vi "Launch CO2 Actor.vi"(4 "SHVs":cluster{"Halt":refnum<k21>}, 5 "DedicatedEnQrs":refnum<queue>, 6 "Open Actor Core front panel? (F)":bool, 7 "Name":string, 8 "error in (no error)":errorcluster, 9 "Interlock Chain":refnum<class "Interlock Chain.lvclass">, 10 "Caller Actor in":refnum<class "Actor.lvclass">, 11 "CO2 Actor in":refnum<class "CO2 Actor.lvclass">) -> (0 "error out":errorcluster, 3 "Caller-To-Actor Enqueuer":refnum<class "Message Enqueuer.lvclass">)   [LabVIEW 2015, in "cRIO-Carbondioxide.lvlib" / "CO2-Actor.lvlib" / "CO2 Actor.lvclass"]
uses:
  CO2 Actor.lvclass
  Interlocks/Interlock Chain/Interlock Chain.lvclass
  <vilib>/ActorFramework/Actor/Actor.lvclass
  <vilib>/ActorFramework/Message Enqueuer/Message Enqueuer.lvclass
  Controls/Dedicated Enqueuers.ctl
  CO2 Actor.lvclass/CO2 Actor.ctl
panel:
  out "CO2 Actor out":refnum<class "CO2 Actor.lvclass">
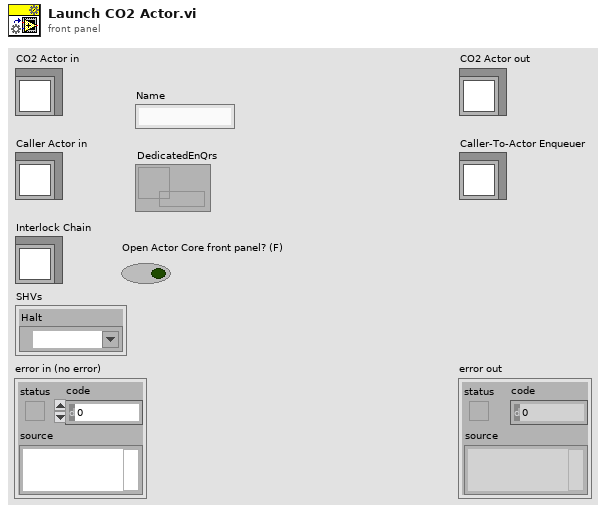
[diagram p1: front panel]
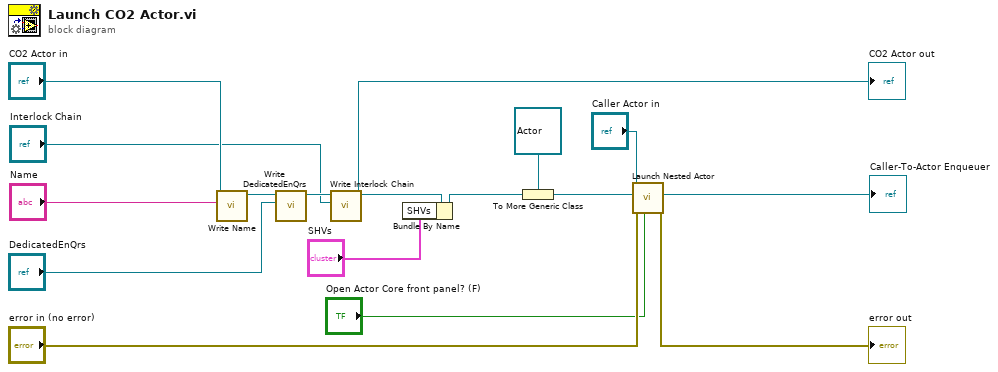
[diagram p0: block diagram]
diagram:
  n1 = call "Write Name.vi"("Name"="Name", "CO2 Actor in"="CO2 Actor in") -> ("CO2 Actor out"=w6:refnum<class "CO2 Actor.lvclass">)  [unwired: 9 in]
  n2 = call "Write DedicatedEnQrs.vi"("DedicatedEnQrs"="DedicatedEnQrs", "CO2 Actor in"=w6) -> ("CO2 Actor out"=w5:refnum<class "CO2 Actor.lvclass">)  [unwired: 9 in]
  n3 = call "Write Interlock Chain.vi"("Interlock Chain"="Interlock Chain", "CO2 Actor in"=w5) -> ("CO2 Actor out"=w13:refnum<class "CO2 Actor.lvclass">)  [unwired: 8 in, 1 out]
  "CO2 Actor out" <- w13
  n4 = Bundle By Name(cluster=w13, "SHVs"="SHVs") -> (w2:refnum<class "CO2 Actor.lvclass">)
  n5 = To More Generic Class(target class=refnum<class "Actor.lvclass"> refnum ("Actor"), reference=w2) -> (generic class reference=w8:refnum<class "Actor.lvclass">)
  n6 = call <vilib>:"Launch Nested Actor.vi"("Open Actor Core front panel? (F)"="Open Actor Core front panel? (F)", "error in (no error)"="error in (no error)", "Nested Actor"=w8, "Caller Actor in"="Caller Actor in") -> ("error out"=→"error out":errorcluster, "Nested Actor's Enqueuer"=→"Caller-To-Actor Enqueuer":refnum<class "Message Enqueuer.lvclass">)  [unwired: 5 in, 1 out]
